vi "LSPOneStatus (SubVI).vi"(11 "VISA Refnum in":refnum<visa-resource-name>) -> (3 "read buffer":string)   [LabVIEW 2020]
panel:
  out "error out":errorcluster
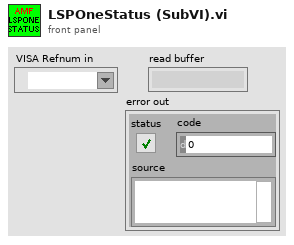
[diagram p1: front panel]
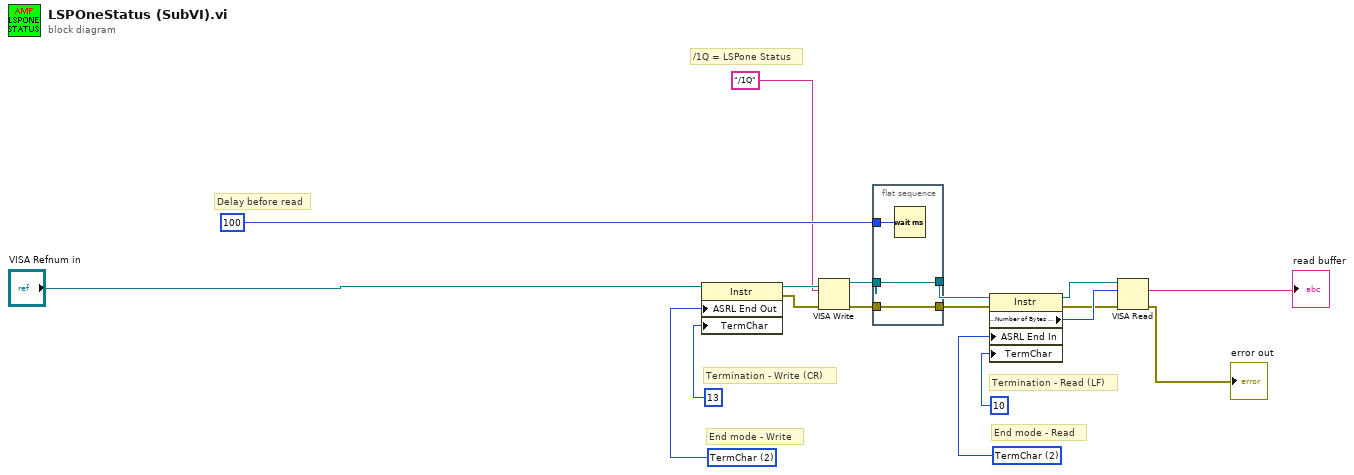
[diagram p0: block diagram]
diagram:
  w17 = u16 2 items=["None", "Last Bit", "TermChar"] ("Serial Settings:End Mode for Reads")
  w14 = u16 2 items=["None", "Last Bit", "TermChar", "Break"] ("Serial Settings:End Mode for Writes")
  # "/1Q = LSPone Status"
  # "End mode - Read"
  # "Termination - Read (LF)"
  # "End mode - Write"
  # "Termination - Write (CR)"
  # "Delay before read"
  n1 = property class="Instr"(reference="VISA Refnum in", "ASRL End Out"=w14, "TermChar"=u8 13 ("Message Based Settings:Termination Character")) -> (reference out=w11:refnum<visa-resource-name>, error out=w12:errorcluster)  [unwired: 1 in]
  n2 = VISA Write(VISA resource name=w11, write buffer="/1Q", error in (no error)=w12) -> (VISA resource name out=w7:refnum<visa-resource-name>, error out=w5:errorcluster)  [unwired: 1 out]
  n3 = flat-sequence {
    tunnel: w5 -> [w20]
    tunnel: [w20] -> w6
    tunnel: w7 -> [w19]
    tunnel: [w19] -> w13
    tunnel: u32 100 ("delay before read (ms)") -> [w21]
    frame #0 {
      n4 = Wait (ms)(milliseconds to wait=w21) -> ()  [unwired: 1 out]
    }
  }
  n5 = property class="Instr"(reference=w13, error in=w6, "ASRL End In"=w17, "TermChar"=u8 10 ("Message Based Settings:Termination Character")) -> (reference out=w2:refnum<visa-resource-name>, error out=w9:errorcluster, "Serial Settings:Number of Bytes at Serial Port"=w10:u32)
  n6 = VISA Read(VISA resource name=w2, byte count=w10, error in (no error)=w9) -> (read buffer=→"read buffer":string, error out=→"error out":errorcluster)  [unwired: 2 out]
